vi "DPad Value To Enum.vi"(10 "D-Pad Value":i32) -> (2 "D-Pad":T1)   [LabVIEW 2011, in "LMH-PS4.lvlib"]
uses:
  LMH-PS4.lvlib
  Type Defs/DpadEnum.ctl
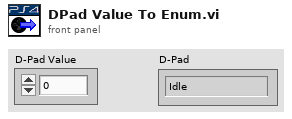
[diagram p1: front panel]
types:
  T1 = typedef "DpadEnum.ctl" = enum16{"Idle", "Up", "Up / Right", "Right", "Down / Right", "Down", "Down / Left", "Left", "Up / Left"}
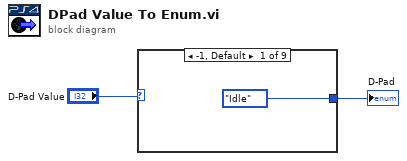
[diagram p0: block diagram]
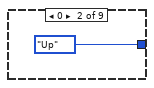
[diagram p2: hidden frame]
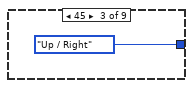
[diagram p3: hidden frame]
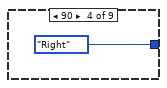
[diagram p4: hidden frame]
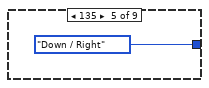
[diagram p5: hidden frame]
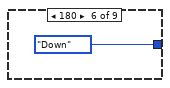
[diagram p6: hidden frame]
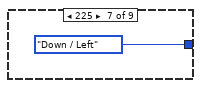
[diagram p7: hidden frame]
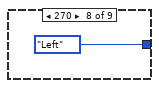
[diagram p8: hidden frame]
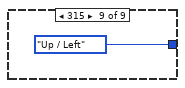
[diagram p9: hidden frame]
diagram:
  n1 = case shown="-1, Default" "D-Pad Value" {
    tunnel: [DpadEnum."Idle" ("D-Pad") DpadEnum."Up" ("D-Pad") DpadEnum."Up / Right" ("D-Pad") DpadEnum."Right" ("D-Pad") DpadEnum."Down / Right" ("D-Pad") DpadEnum."Down" ("D-Pad") DpadEnum."Down / Left" ("D-Pad") DpadEnum."Left" ("D-Pad") DpadEnum."Up / Left" ("D-Pad")] -> w1
    frame -1, Default {
    }
    frame 0 {
    }
    frame 45 {
    }
    frame 90 {
    }
    frame 135 {
    }
    frame 180 {
    }
    frame 225 {
    }
    frame 270 {
    }
    frame 315 {
    }
  }
  "D-Pad" <- w1
